vi "Draw Circle 2015 NIVerified.vi"() -> ()   [LabVIEW 2015]
panel:
  in  "Y Origin":dbl
  in  "X Origin":dbl
  in  "Magnitude":dbl
  in  "Number of Points":i32=200
  out "XY Graph":cluster{dbl[], dbl[]}(graph)
  # "Overview: This VI Draws a circle in an XY Graph.\nRequirements: LabVIEW Full Development System.\nInstructions:\n1. Fill in the reguired Magnitude and Number of points.\n2. Use the X Origin and Y Origin to define the centre of the circle.\n2. Run the program."
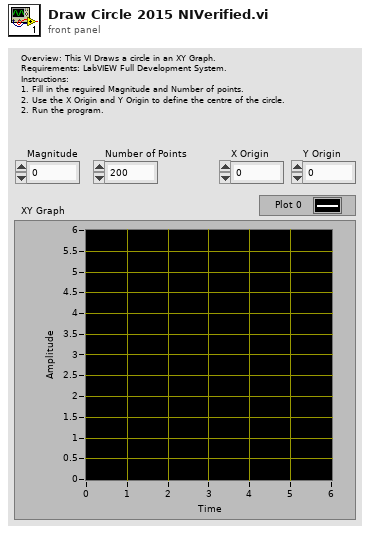
[diagram p1: front panel]
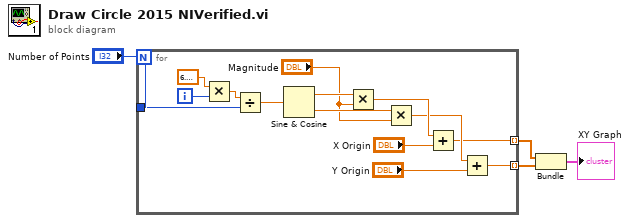
[diagram p0: block diagram]
diagram:
  n1 = for {
    N: "Number of Points" -> [_]
    tunnel: "Number of Points" -> [w16]
    tunnel: [w6] -> w1 mode=indexing
    tunnel: [w5] -> w2 mode=indexing
    i -> [w18]
    n2 = Multiply(x=6.283185307179586, y=w18) -> (x*y=w17:dbl)
    n3 = Divide(x=w17, y=w16) -> (x/y=w14:dbl)
    n4 = Sine & Cosine(0:w14) -> (1:w13:dbl, 2:w12:dbl)
    n5 = Multiply(x=w13, y="Magnitude") -> (x*y=w10:dbl)
    n6 = Multiply(x=w12, y="Magnitude") -> (x*y=w9:dbl)
    n7 = Add(x=w10, y="X Origin") -> (x+y=w6:dbl)
    n8 = Add(x=w9, y="Y Origin") -> (x+y=w5:dbl)
  }
  n9 = Bundle(w1, w2) -> (→"XY Graph":cluster{dbl[], dbl[]})  [unwired: 1 in]
